vi "Var_globale.vi"() -> ()   [LabVIEW 2009]
panel:
  in  "K1":bool
  in  "N1":dbl
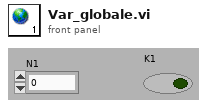
[diagram p1: front panel]
diagram:
